vi "make 2d scan file with drift check.vi"() -> ()   [LabVIEW 2013]
uses:
  scan parameters.ctl
panel:
  in  "check value":dbl
  in  "start scan":i32
  in  "precision (12)":i16=12
  in  "reverse which par is scanned":bool
  in  "2D scan details":T2(array[cluster])=[{"Scan parameters"={"Scan Start"=1.1e-06, "Scan End"=2.1e-06, "Scan Step Size"=5e-08, "# Shots Each Step"=7, "single direction?"=TRUE}, "device and variable preamble"="Device = \"HeatHighlandT564\"\nVariable = \"Discharge timing s\""}, {"Scan parameters"={"Scan Start"=10.0, "Scan End"=70.0, "Scan Step Size"=5.0, "# Shots Each Step"=1, "single direction?"=TRUE}, "device and variable preamble"="Device = \"PL1-PresCtrl-Low1\"\nVariable = \"P. Control Down (Torr)\""}] {"Scan parameters"."Scan Start" format="%#.9p"; "Scan parameters"."Scan End" format="%#.9p"; "Scan parameters"."Scan Step Size" format="%#.9p"}
  out "spreadsheet string":string
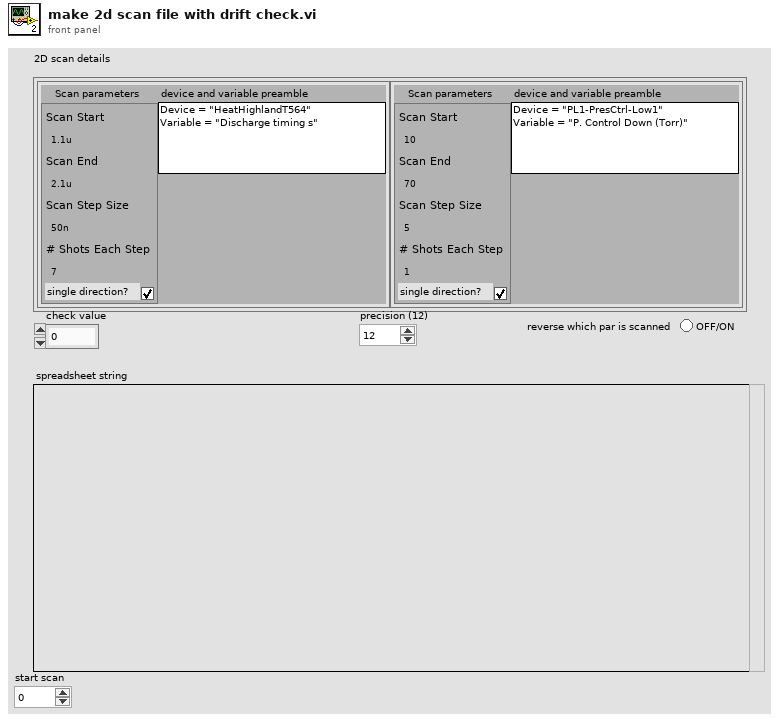
[diagram p1: front panel]
types:
  T1 = typedef "scan parameters.ctl" = cluster{"Scan Start":dbl, "Scan End":dbl, "Scan Step Size":dbl, "# Shots Each Step":u32, "single direction?":bool}
  T2 = cluster{"Scan parameters":T1, "device and variable preamble":string}[]
  T3 = cluster{"Scan parameters":T1, "device and variable preamble":string}
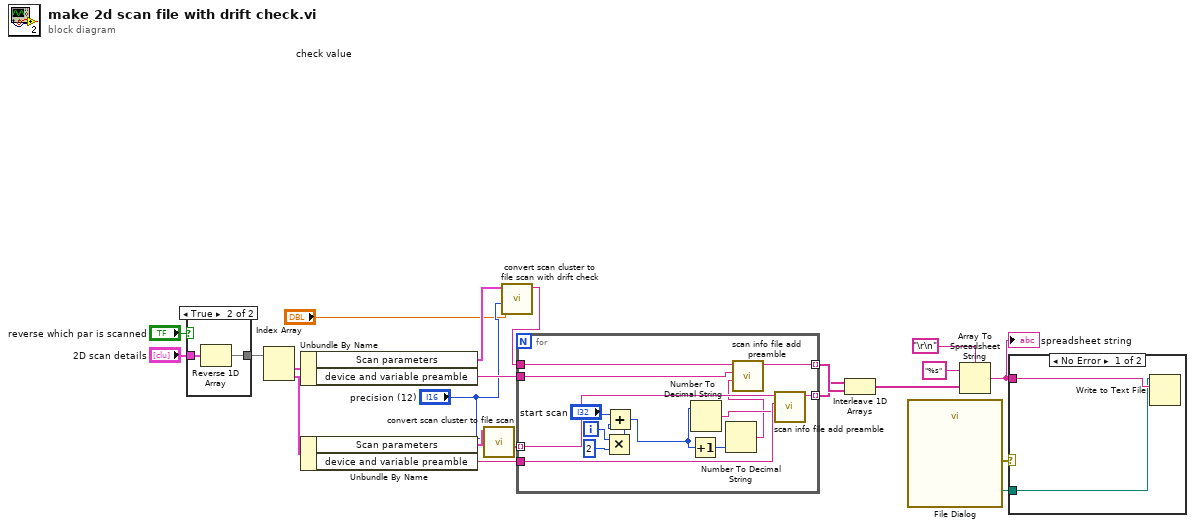
[diagram p0: block diagram]
diagram:
  n1 = case shown="True" "reverse which par is scanned" {
    tunnel: "2D scan details" -> [w22 w24]
    tunnel: [w22 w23] -> w10
    frame False {
    }
    frame True {
      n2 = Reverse 1D Array(array=w24) -> (reversed array=w23:T2)
    }
  }
  n3 = Index Array(array=w10) -> (element #1=w8:T3, element #2=w7:T3)  [unwired: 2 in]
  n4 = Unbundle By Name(w8) -> ("Scan parameters"=w4:T1, "device and variable preamble"=w12:string)
  n5 = Unbundle By Name(w7) -> ("Scan parameters"=w6:T1, "device and variable preamble"=w5:string)
  n6 = call "convert scan cluster to file scan.vi"("precision (12)"="precision (12)", "Scan parameters"=w6) -> ("values:numshots"=w18:string[])  [unwired: 7 in, 2 out]
  n7 = call "convert scan cluster to file scan with drift check.vi"("Scan parameters"=w4, "check value"="check value", "precision (12)"="precision (12)") -> ("spreadsheet string"=w1:string)  [unwired: 5 in, 2 out]
  n8 = for {
    tunnel: [w36] -> w19 mode=indexing
    tunnel: w1 -> [w37]
    tunnel: w18 -> [w34] mode=indexing
    tunnel: [w33] -> w16 mode=indexing
    tunnel: w12 -> [w32]
    tunnel: w5 -> [w31]
    i -> [w28]
    n9 = Multiply(x=w28, y=2) -> (x*y=w27:i32)
    n10 = Add(x="start scan", y=w27) -> (x+y=w25:i32)
    n11 = Increment(x=w25) -> (x+1=w35:i32)
    n12 = Number To Decimal String(number=w25) -> (decimal integer string=w30:string)  [unwired: 1 in]
    n13 = Number To Decimal String(number=w35) -> (decimal integer string=w29:string)  [unwired: 1 in]
    n14 = call "scan info file add preamble.vi"("scan #"=w29, "device and variable stuff"=w32, "spreadsheet string"=w37) -> ("scan text for txt file"=w36:string)  [unwired: 8 in]
    n15 = call "scan info file add preamble.vi"("scan #"=w30, "device and variable stuff"=w31, "spreadsheet string"=w34) -> ("scan text for txt file"=w33:string)  [unwired: 8 in]
  }
  n16 = Interleave 1D Arrays(w16, w19) -> (w17:string[])
  n17 = call "File Dialog"() -> ("selected path"=w13:path, "error out"=w14:errorcluster)  [unwired: 12 in, 2 out]
  n18 = Array To Spreadsheet String(delimiter (Tab)="\r\n", array=w17, 3:"%s" ("format string")) -> (spreadsheet string=w15:string)
  "spreadsheet string" <- w15
  n19 = case shown="No Error" w14 {
    tunnel: w15 -> [w40 _]
    tunnel: w13 -> [w39 _]
    frame No Error {
      n20 = Write to Text File(file (use dialog)=w39, text=w40) -> ()  [unwired: 2 in, 3 out]
    }
    frame Error {
    }
  }
